vi "Verify CLI Output.vi"(5 "Label":string, 7 "Approval Tests.lvlib:Options.lvclass":refnum<class "Options.lvclass">, 8 "error in":errorcluster, 9 "CLI Options":T1={"standard input"="", "working directory"=path "", "expected output size  (4096)"=4096, "Run Minimized (T)"=TRUE}, 10 "command line":string) -> (0 "error out":errorcluster, 1 "Failure Message":string, 2 "Passed?":bool)   [LabVIEW 2020, in "Approval Tests.lvlib"]
doc: "Uses System Exec to execute command.\n\nCaptures:\nSTD out\nERR out\nReturn Code"
uses:
  Approval Tests.lvlib
  Options/Options.lvclass
  Verify CLI Options.ctl
  Options/Options.lvclass/Options.ctl
  Naming Data/Naming Data.lvclass/Naming Data.ctl
  a806700d-e4e9-4561-ab5d-90979b88ac20.vi
  Naming Data/Read Test VI Name.vi
  Naming Data/Write Test VI Name.vi
  Verify Core.vi
  a806700d-e4e9-4561-ab5d-90979b88ac20.vi/93c5622b-9fb7-41e0-8c76-3fde37e94e34.vi
  Options/Read Scrubber.vi
  Options/Read Namer.vi
  Options/Read Naming Data.vi
  Options/Read Reporter.vi
  Options/Read Text Comparator.vi
  a806700d-e4e9-4561-ab5d-90979b88ac20.vi/93c5622b-9fb7-41e0-8c76-3fde37e94e34.vi/04cb982b-2eda-40d0-8d7e-90f8e0b569b2.vi
  a806700d-e4e9-4561-ab5d-90979b88ac20.vi/93c5622b-9fb7-41e0-8c76-3fde37e94e34.vi/04cb982b-2eda-40d0-8d7e-90f8e0b569b2.vi/04ec6d97-7b7c-4123-b264-4b7eb8a41208.vi
  <vilib>/PNR/JSONtext Object Serialization/Generic Object Serializer/Generic Object Serializer.lvclass
  C:/Program Files/National Instruments/LabVIEW 2026/vi.lib/JDP Science/JSONtext/LVClass Serializer/JSONtext LVClass Serializer.lvclass
  Options/Add Label to Namer.vi
  <vilib>/JDP Science/JSONtext/Variant to JSON Text.vi
  conv EOL.vi
  <vilib>/Utility/libraryn.llb/Check if File or Folder Exists.vi
  Reporter/Report.vi
  Scrubber/Scrubber.lvclass
  Namer/Namer.lvclass
  Naming Data/Naming Data.lvclass
  Reporter/Reporter.lvclass
  Text Comparator/Text Comparator.lvclass
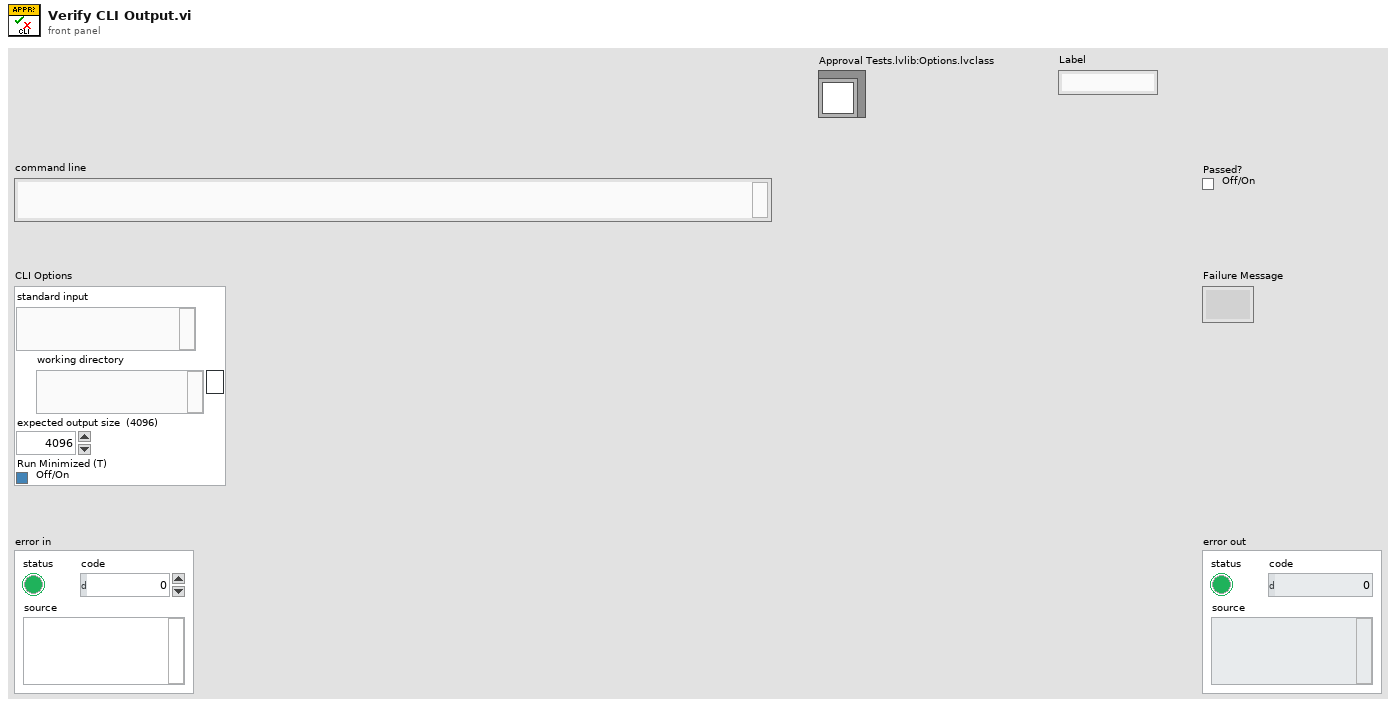
[diagram p1: front panel]
types:
  T1 = typedef "Approval Tests.lvlib/Verify CLI Options.ctl" = cluster{"standard input":string, "working directory":path, "expected output size  (4096)":u32, "Run Minimized (T)":bool}
  T2 = cluster{"standard output":string, "standard error":string, "return code":i32}
  T3 = enum16{"Native", "Native Command Line", "UNIX", "Macintosh", "DOS"}
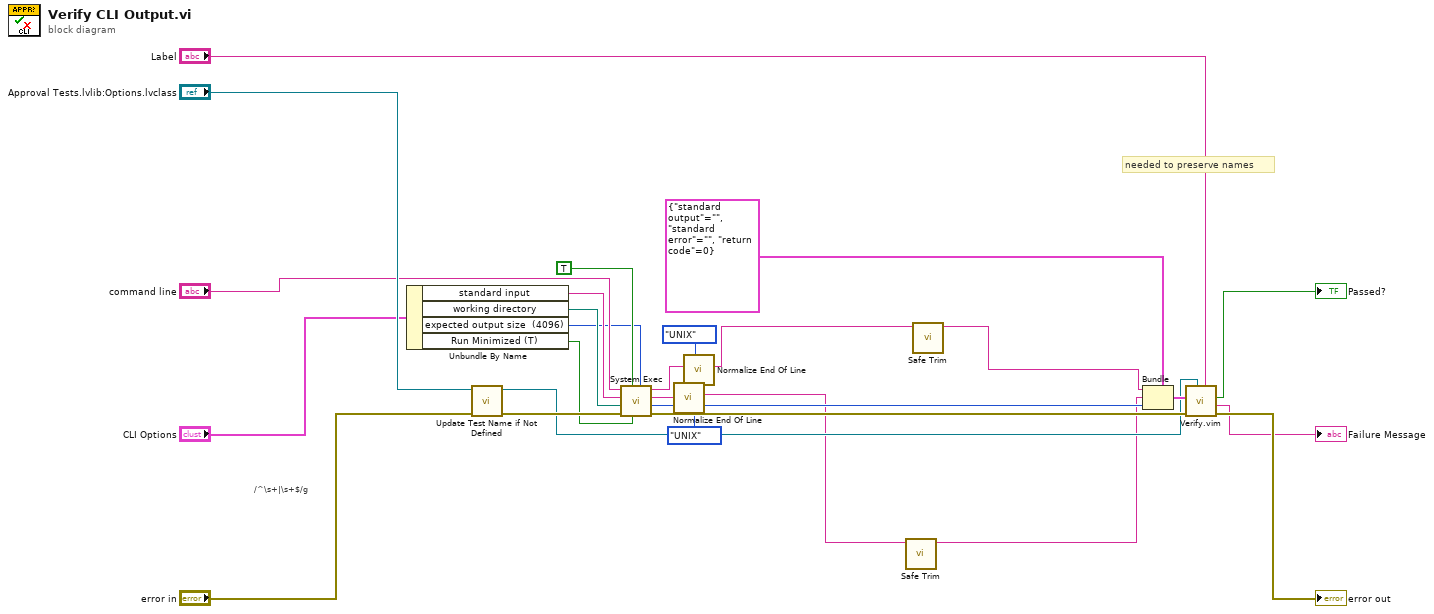
[diagram p0: block diagram]
diagram:
  # "/^\\s+|\\s+$/g"
  # "needed to preserve names"
  n1 = Unbundle By Name("CLI Options") -> ("standard input"=w13:string, "working directory"=w12:path, "expected output size  (4096)"=w11:u32, "Run Minimized (T)"=w14:bool)
  n2 = call "Update Test Name if Not Defined.vi"("error in"="error in", "Options in"="Approval Tests.lvlib:Options.lvclass") -> ("error out"=w25:errorcluster, "Options out"=w18:refnum<class "Options.lvclass">)  [unwired: 8 in]
  n3 = call <vilib>:"System Exec.vi"("expected output size  (4096)"=w11, "run minimized? (F)"=w14, "wait until completion? (T)"=TRUE, "error in (no error)"=w25, "working directory"=w12, "standard input"=w13, "command line"="command line") -> ("error out"=w24:errorcluster, "return code"=w20:i32, "standard error"=w10:string, "standard output"=w9:string)  [unwired: 1 in]
  n4 = call <vilib>:"Normalize End Of Line.vi"("end of line (Native)"=T3."UNIX", "string in"=w10) -> ("string out"=w4:string)  [unwired: 6 in]
  n5 = call <vilib>:"Normalize End Of Line.vi"("end of line (Native)"=T3."UNIX", "string in"=w9) -> ("string out"=w2:string)  [unwired: 6 in]
  n6 = call "Safe Trim.vi"("string in"=w4) -> ("result string"=w3:string)  [unwired: 10 in]
  n7 = call "Safe Trim.vi"("string in"=w2) -> ("result string"=w1:string)  [unwired: 10 in]
  n8 = Bundle(cluster=T2 {"standard output"="", "standard error"="", "return code"=0}, "standard output"=w1, "standard error"=w3, "return code"=w20) -> (w19:T2)
  n9 = call "Verify.vim"("Label"="Label", "Options"=w18, "error in"=w24, "Anything"=w19) -> ("error out"=→"error out":errorcluster, "Failure Message"=→"Failure Message":string, "Passed?"=→"Passed?":bool)  [unwired: 5 in]
